vi "Cascade MEMS Only Gen0 VCmin.vi"(7 "V Bias":dbl, 8 "Error In":errorcluster, 9 "V3":string[](array[string]), 10 "V2":string[](array[string]), 11 "V1":string[](array[string])) -> (0 "Error Out":errorcluster, 3 "VCmin":string[](array[string]))   [LabVIEW 2017]
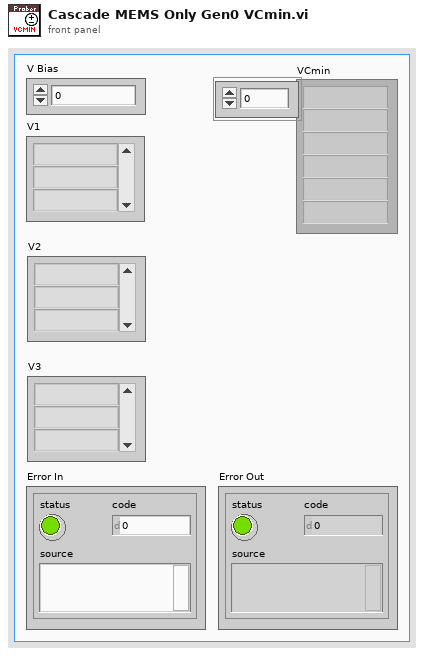
[diagram p1: front panel]
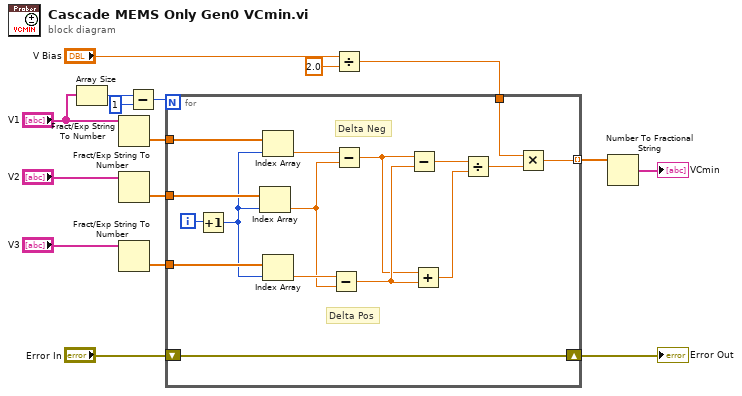
[diagram p0: block diagram]
diagram:
  n1 = Array Size(array="V1") -> (size(s)=w2:i32)
  n2 = Fract/Exp String To Number(string="V1") -> (number=w14:dbl[])  [unwired: 3 in, 1 out]
  n3 = Fract/Exp String To Number(string="V2") -> (number=w12:dbl[])  [unwired: 3 in, 1 out]
  n4 = Fract/Exp String To Number(string="V3") -> (number=w13:dbl[])  [unwired: 3 in, 1 out]
  n5 = Subtract(x=w2, y=1) -> (x-y=w3:i32)
  n6 = Divide(x="V Bias", y=2.0) -> (x/y=w9:dbl)
  n7 = for {
    N: w3 -> [_]
    tunnel: w14 -> [w32]
    tunnel: w13 -> [w31]
    tunnel: w12 -> [w29]
    tunnel: w9 -> [w21]
    tunnel: [w18] -> w8 mode=indexing
    shift-right: [w17] -> w5
    shift-left: "Error In" -> [w17]
    i -> [w20]
    # "Delta Pos"
    # "Delta Neg"
    n8 = Increment(x=w20) -> (x+1=w19:i32)
    n9 = Index Array(array=w29, index=w19) -> (element=w27:dbl)
    n10 = Index Array(array=w32, index=w19) -> (element=w30:dbl)
    n11 = Index Array(array=w31, index=w19) -> (element=w28:dbl)
    n12 = Subtract(x=w28, y=w27) -> (x-y=w26:dbl)
    n13 = Subtract(x=w30, y=w27) -> (x-y=w25:dbl)
    n14 = Subtract(x=w25, y=w26) -> (x-y=w24:dbl)
    n15 = Add(x=w25, y=w26) -> (x+y=w23:dbl)
    n16 = Divide(x=w24, y=w23) -> (x/y=w22:dbl)
    n17 = Multiply(x=w21, y=w22) -> (x*y=w18:dbl)
  }
  "Error Out" <- w5
  n18 = Number To Fractional String(number=w8) -> (F-format string=→"VCmin":string[])  [unwired: 3 in]
